vi "EditVIPBPackageVersion.vi"(7 "package version":string, 8 "error in":errorcluster, 11 "path to vipb file":path) -> (0 "error out":errorcluster)   [LabVIEW 2019]
uses:
  <vilib>/JKI/VIPM API/VIPM API_vipm_api.lvlib
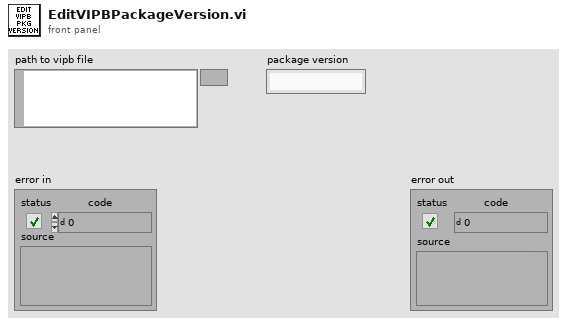
[diagram p1: front panel]
types:
  T1 = typedef "VIPM API_vipm_api.lvlib/VI Package Build Spec Data Cluster_vipm_api.ctl" = cluster{"Package Version":T2, "Product Name":string, "Company Name":string, "Author Name (Person or Company)":string, "Product Homepage (URL)":string, "Legal Copyright":string, "License Agreement Name":string, "Product Description Summary":string, "Product Description":string, "Release Notes - Change Log":string}
  T2 = typedef "VIPM API_vipm_api.lvlib/Version Info Cluster_vipm_api.ctl" = cluster{"major":u32, "minor":u32, "patch":u32, "build":u32}
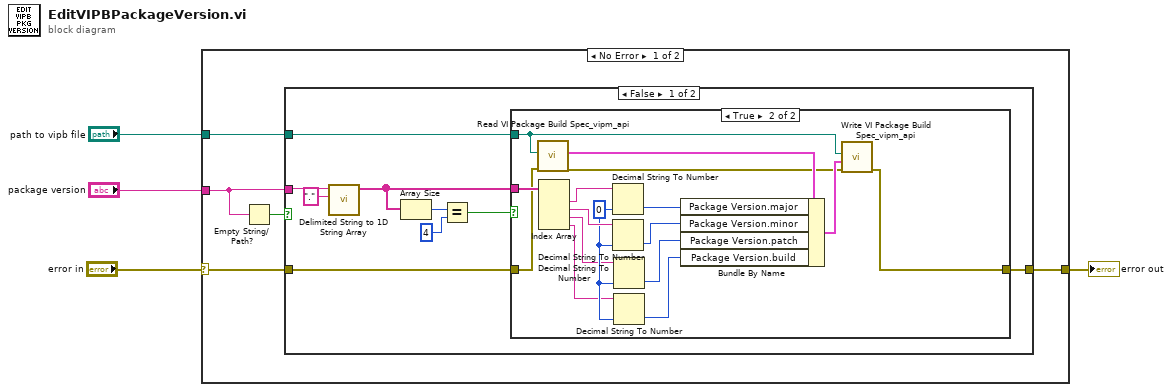
[diagram p0: block diagram]
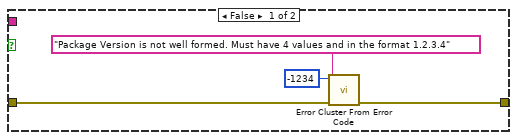
[diagram p2: hidden frame]
diagram:
  n1 = case shown="No Error" "error in" {
    selector: "error in" -> [w7 w40]
    tunnel: "path to vipb file" -> [w5 _]
    tunnel: [w6 w40] -> w2
    tunnel: "package version" -> [w8 _]
    frame No Error {
      n2 = Empty String/Path?(string/path=w8) -> (empty?=w9:bool)
      n3 = case shown="False" w9 {
        tunnel: w8 -> [w15 _]
        tunnel: w7 -> [w12 w39]
        tunnel: [w11 w39] -> w6
        tunnel: w5 -> [w10 _]
        frame False {
          n4 = call <vilib>:"Delimited String to 1D String Array.vi"("delimiter"=".", "delimited string"=w15) -> ("string array"=w13:string[])  [unwired: 9 in]
          n5 = Array Size(array=w13) -> (size(s)=w18:i32)
          n6 = Equal?(x=w18, y=4) -> (x = y?=w14:bool)
          n7 = case shown="True" w14 {
            tunnel: w13 -> [_ w37]
            tunnel: w12 -> [w20 w36]
            tunnel: [w19 w23] -> w11
            tunnel: w10 -> [_ w26]
            frame False {
              n8 = call <vilib>:"Error Cluster From Error Code.vi"("error in (no error)"=w20, "error message (\"\")"="Package Version is not well formed. Must have 4 values and in the format 1.2.3.4" ("error message (\"\")"), "error code (0)"=-1234) -> ("error out"=w19:errorcluster)  [unwired: 6 in]
            }
            frame True {
              w33 = u32 0 ("Package Version.major")
              n9 = call <vilib>:"Read VI Package Build Spec_vipm_api.vi"("error in (no error)"=w36, "Path to VIPB File"=w26) -> ("error out"=w24:errorcluster, "VI Package Build Spec Data"=w38:T1)  [unwired: 8 in]
              n10 = Index Array(array=w37) -> (element #1=w35:string, element #2=w34:string, element #3=w32:string, element #4=w31:string)  [unwired: 4 in]
              n11 = Decimal String To Number(string=w35, default (0L)=w33) -> (number=w30:u32)  [unwired: 1 in, 1 out]
              n12 = Decimal String To Number(string=w34, default (0L)=w33) -> (number=w29:u32)  [unwired: 1 in, 1 out]
              n13 = Decimal String To Number(string=w32, default (0L)=w33) -> (number=w28:u32)  [unwired: 1 in, 1 out]
              n14 = Decimal String To Number(string=w31, default (0L)=w33) -> (number=w27:u32)  [unwired: 1 in, 1 out]
              n15 = Bundle By Name(cluster=w38, "Package Version.major"=w30, "Package Version.minor"=w29, "Package Version.patch"=w28, "Package Version.build"=w27) -> (w25:T1)
              n16 = call <vilib>:"Write VI Package Build Spec_vipm_api.vi"("error in (no error)"=w24, "VI Package Build Spec Data"=w25, "Path to VIPB File"=w26) -> ("error out"=w23:errorcluster)  [unwired: 8 in]
            }
          }
        }
        frame True {
          # "If empty, do nothing. Leave the VIPB file alone."
        }
      }
    }
    frame Error {
      # "If there is already an error, do not edit the file"
    }
  }
  "error out" <- w2
